vi "Pump_API_ForceMonitoring_Test.vi"() -> ()   [LabVIEW 2010]
uses:
  labbCAN_Bus_API/labbCAN_Bus_API.lvlib
  labbCAN_Pump_API/labbCAN_Pump_API.lvlib
panel:
  out "Force Plot":dbl(graph)
  out "Safety Stop Active":bool
  out "Force":dbl
  out "Flow":dbl
  out "Force Monitoring Enabled":bool
  out "Position Sensing Initialized":bool
  out "Status":string="Test 5: Continuous flow dosage"
  out "Test Step:":string
  out "error out":errorcluster
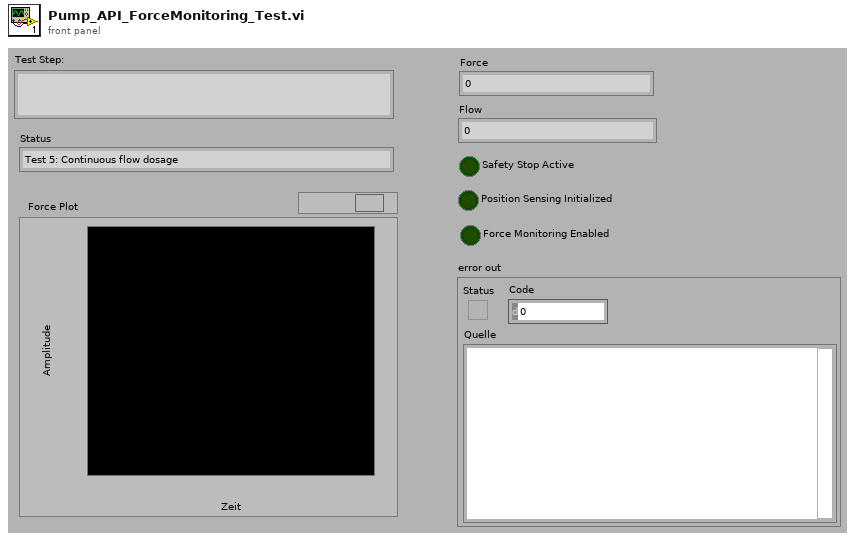
[diagram p1: front panel]
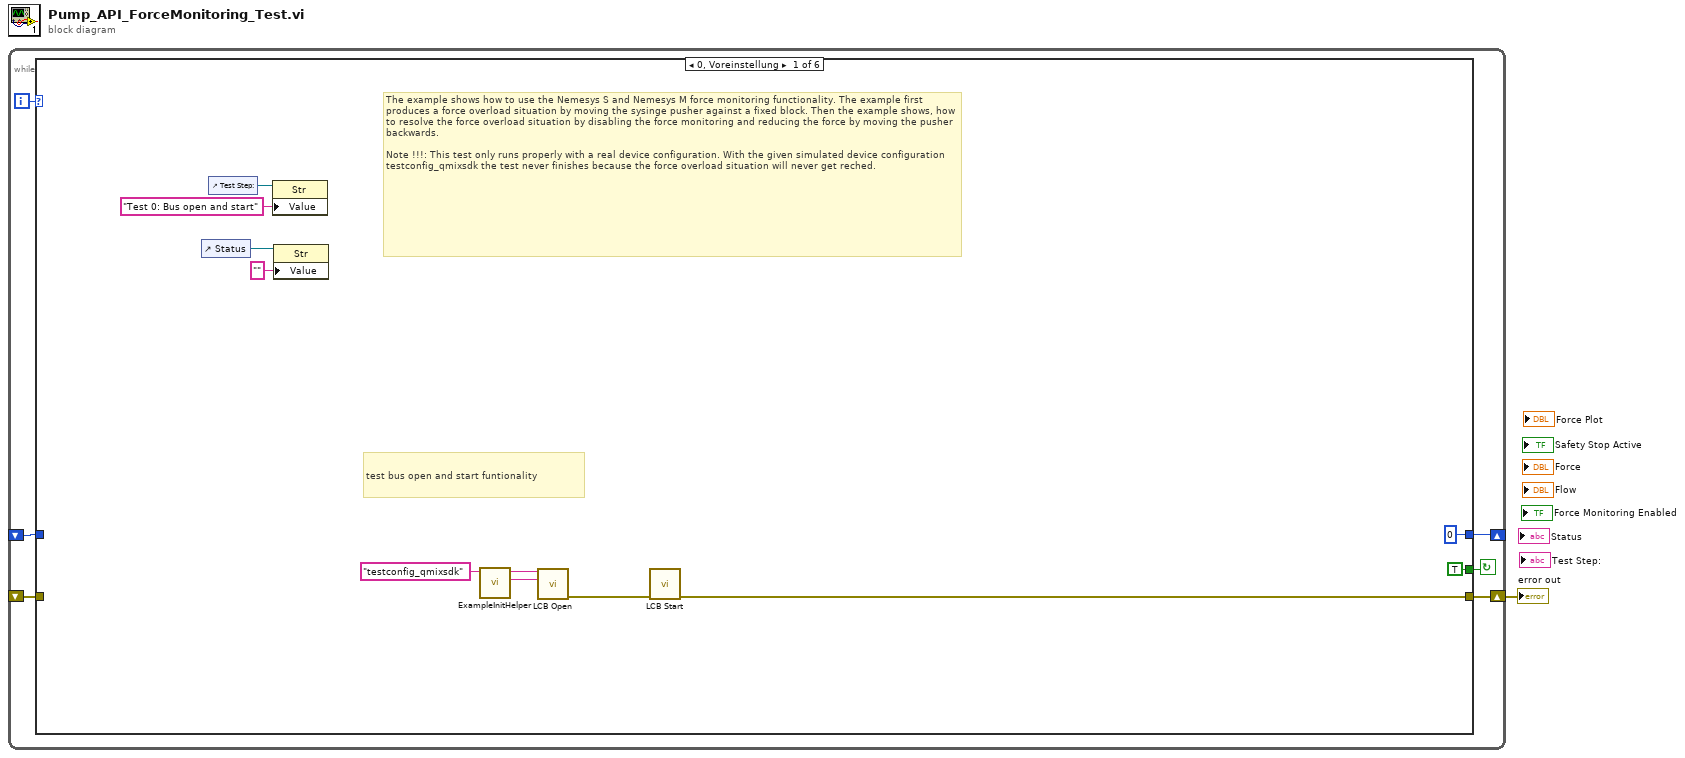
[diagram p0: block diagram]
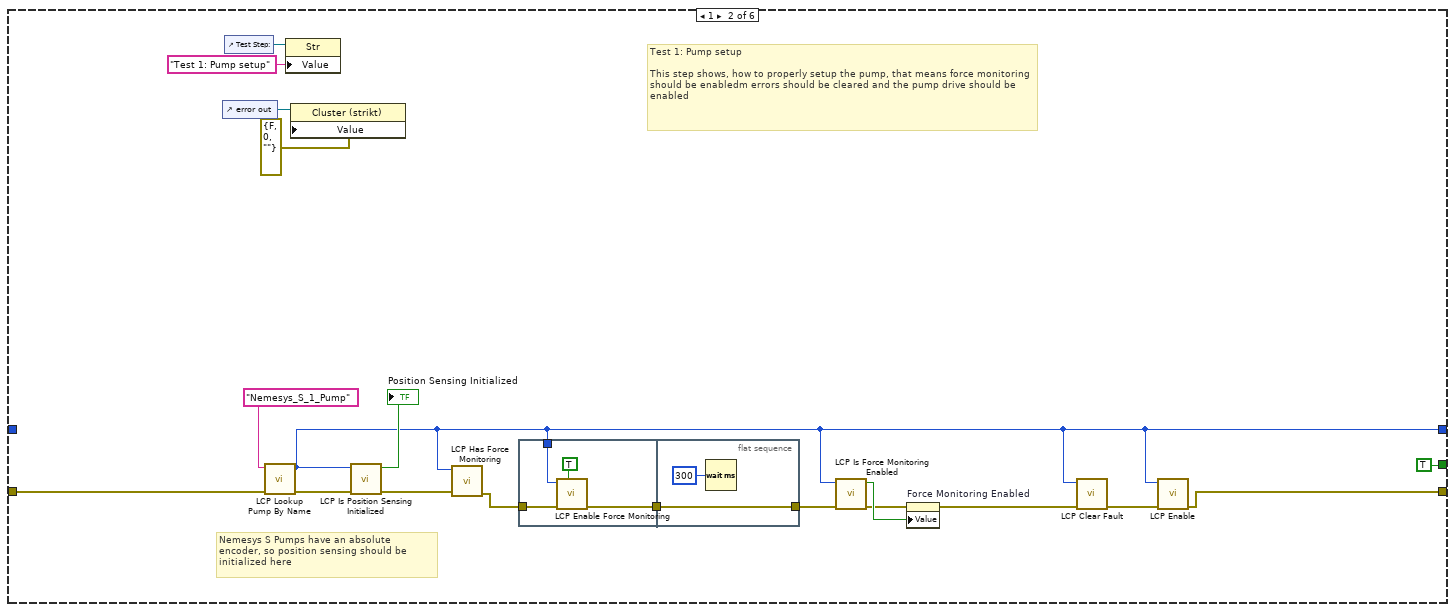
[diagram p2: hidden frame]
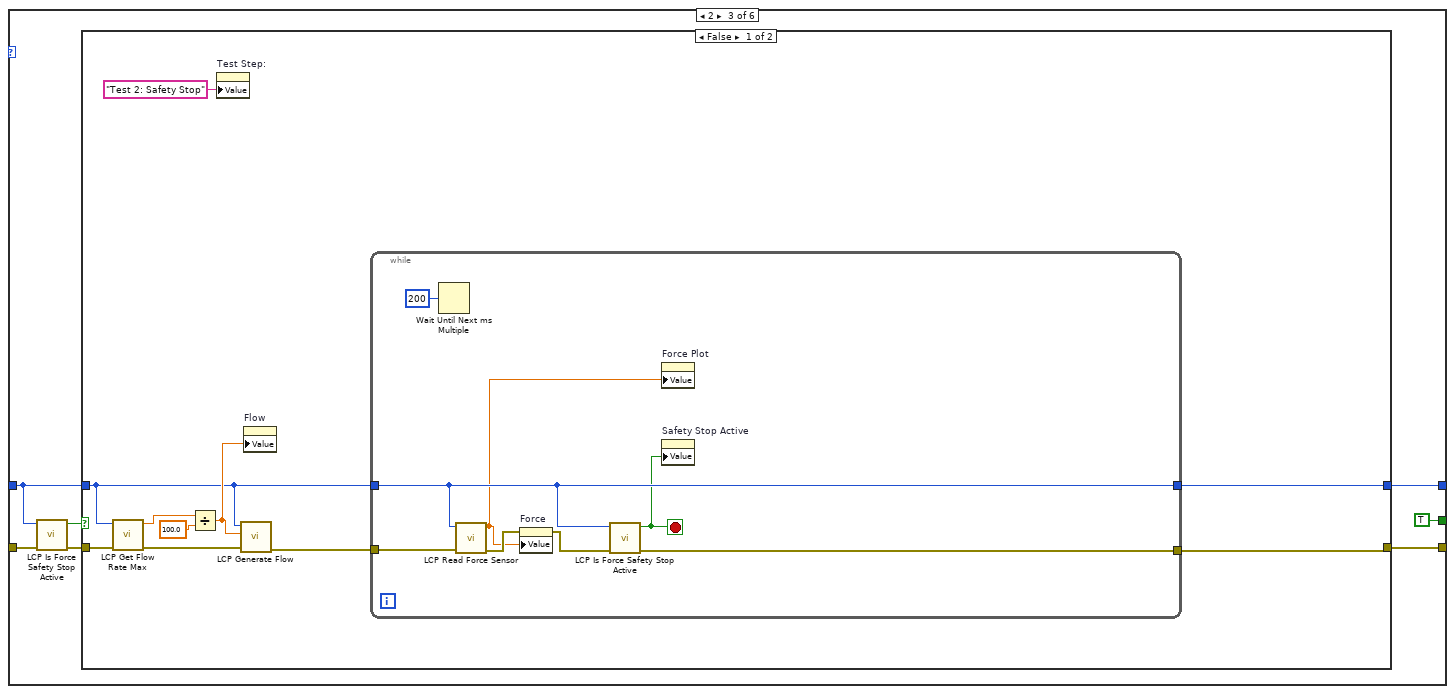
[diagram p3: hidden frame]
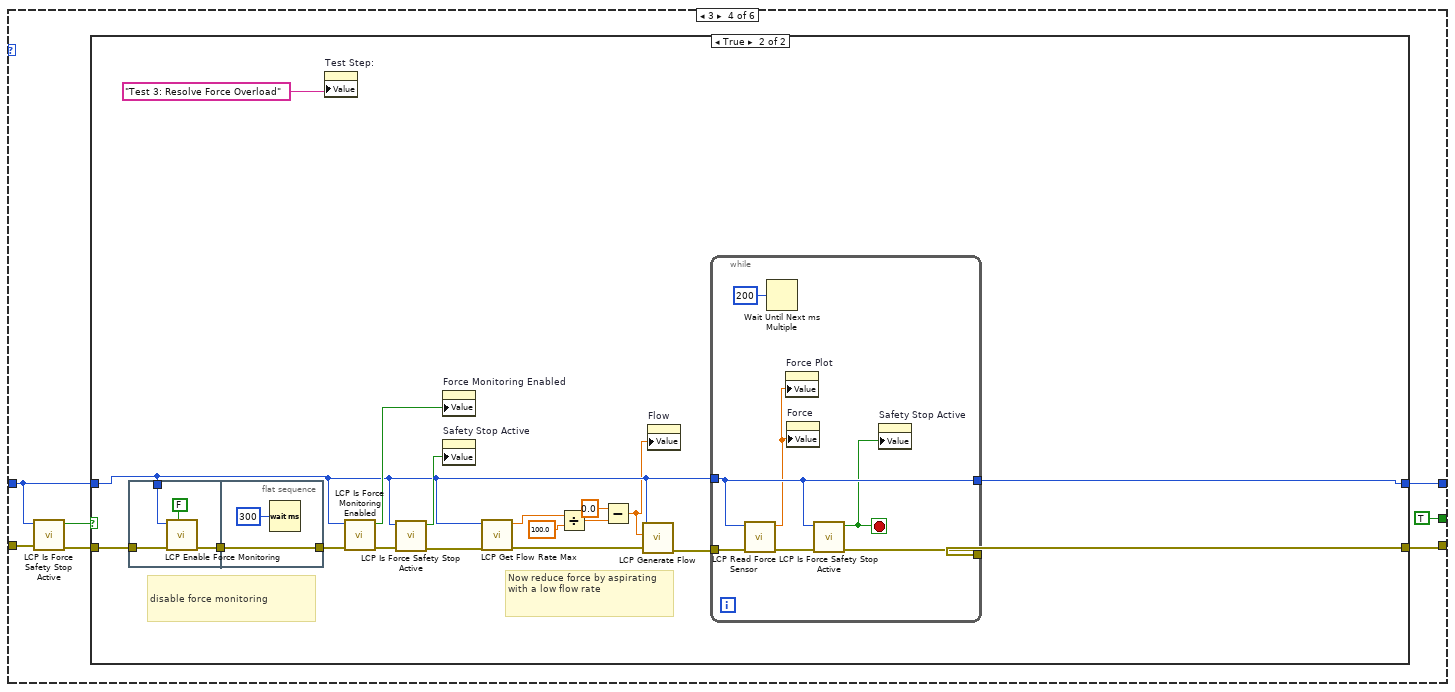
[diagram p5: hidden frame]
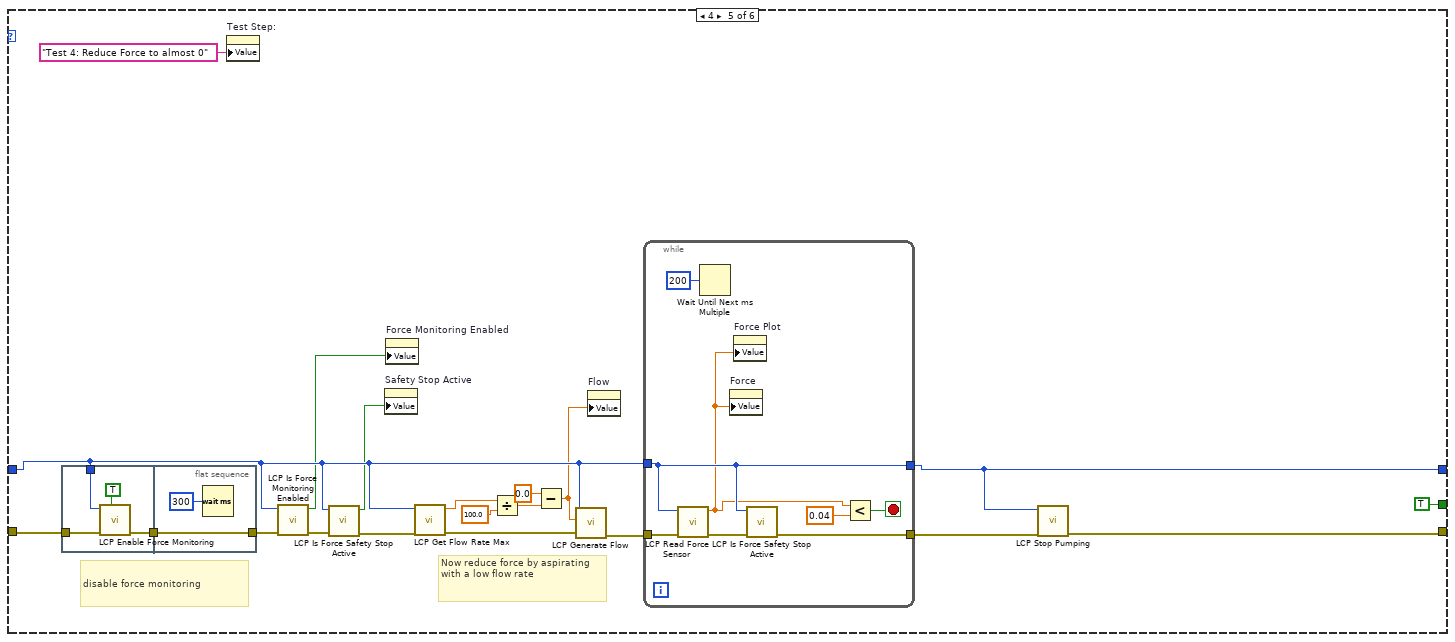
[diagram p7: hidden frame]
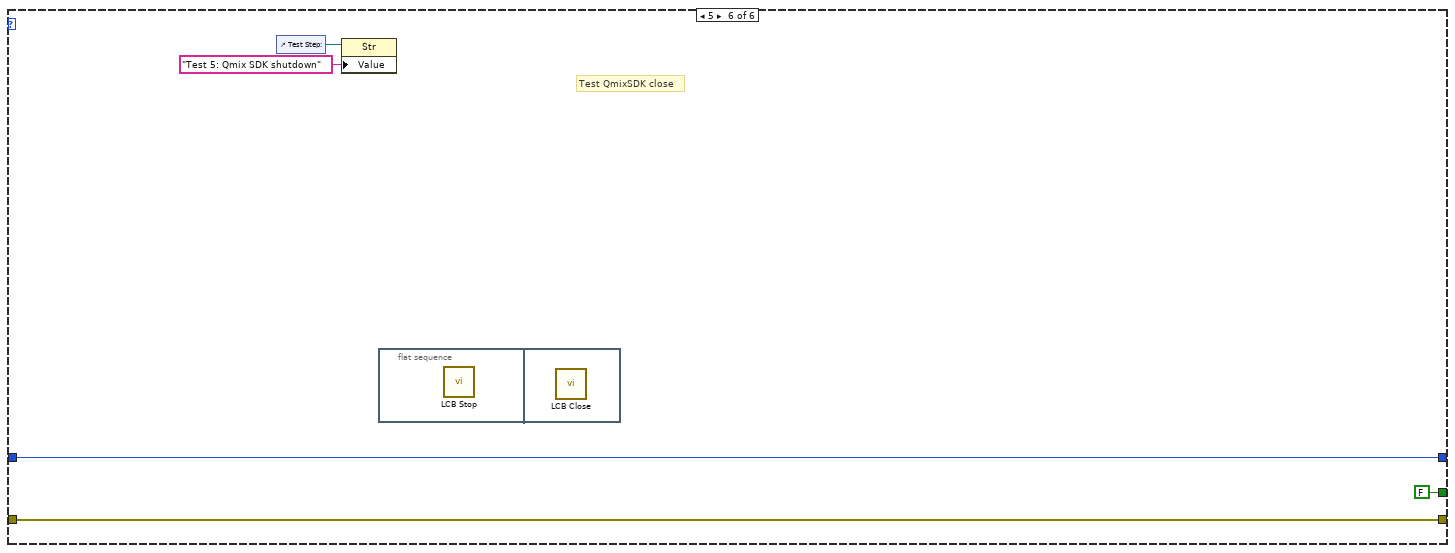
[diagram p8: hidden frame]
diagram:
  n1 = while {
    shift-right: [w2] -> w1
    shift-left: _ -> [w5]
    shift-right: [w4] -> _
    shift-left: _ -> [w3]
    i -> [w7]
    stop <- w6 continue-if-true
    n2 = case shown="0, Voreinstellung" w7 {
      tunnel: [TRUE TRUE TRUE TRUE TRUE FALSE] -> w6
      tunnel: w5 -> [_ w35 w49 w77 w119 w145]
      tunnel: [w16 w19 w46 w75 w112 w145] -> w2
      tunnel: [i64 0 ("ContiFlowPumpHandle") w20 w44 w71 w111 w148] -> w4
      tunnel: w3 -> [_ _ w45 w72 w118 w148]
      frame 0, Default {
        # "The example shows how to use the Nemesys S and Nemesys M force monitoring functionality. The example first produces a force overload situation by moving the sysinge pusher against a fixed block. Then the example shows, how to resolve the force overload situation by disabling the force monitoring and reducing the force by moving the pusher backwards.\n\nNote !!!: This test only runs properly with a real device configuration. With the given simulated device configuration testconfig_qmixsdk the test never finishes because the force overload situation will never get reched."
        # "test bus open and start funtionality"
        n3 = control-ref of="Status"() -> (w12:refnum<vi>)
        n4 = control-ref of="Test Step:"() -> (w14:refnum<vi>)
        n5 = property class="Str"(reference=w14, "Value"="Test 0: Bus open and start" ("Wert")) -> ()  [unwired: 1 in, 2 out]
        n6 = property class="Str"(reference=w12, "Value"="" ("Wert")) -> ()  [unwired: 1 in, 2 out]
        n7 = call "ExampleInitHelper.vi"("Device Config Name"="testconfig_qmixsdk") -> ("Plugin Search Path"=w9:string, "Device Configuration Path"=w10:string)  [unwired: 5 in]
        n8 = call "LCB Open.vi"("PluginSearchPath"=w9, "Device Configuration Path"=w10) -> ("error out"=w17:errorcluster)  [unwired: 9 in]
        n9 = call "LCB Start.vi"("error in (no error)"=w17) -> ("error out"=w16:errorcluster)  [unwired: 10 in]
      }
      frame 1 {
        # "Nemesys S Pumps have an absolute encoder, so position sensing should be initialized here"
        # "Test 1: Pump setup\n\nThis step shows, how to properly setup the pump, that means force monitoring should be enabledm errors should be cleared and the pump drive should be enabled"
        n10 = control-ref of="error out"() -> (w32:refnum<vi>)
        n11 = control-ref of="Test Step:"() -> (w34:refnum<vi>)
        n12 = call "LCP Lookup Pump By Name.vi"("error in (no error)"=w35, "Pump Name"="Nemesys_S_1_Pump" ("pAxisName")) -> ("error out"=w30:errorcluster, "Pump handle"=w20:i64)  [unwired: 8 in]
        n13 = property class="Str"(reference=w34, "Value"="Test 1: Pump setup" ("Wert")) -> ()  [unwired: 1 in, 2 out]
        n14 = property class="Cluster (strikt)"(reference=w32, "Value"=errorcluster {"status"=FALSE, "code"=0, "source"=""} ("Wert")) -> ()  [unwired: 1 in, 2 out]
        n15 = call "LCP Is Position Sensing Initialized.vi"("error in (no error)"=w30, "Pump Handle"=w20) -> ("error out"=w28:errorcluster, "Initialized"=→"Position Sensing Initialized":bool)  [unwired: 8 in]
        n16 = call "LCP Has Force Monitoring.vi"("error in (no error)"=w28, "Pump Handle"=w20) -> ("error out"=w27:errorcluster)  [unwired: 8 in, 1 out]
        n17 = flat-sequence {
          tunnel: w27 -> [w40]
          tunnel: w20 -> [w39]
          tunnel: [w38] -> w26
          tunnel: [w42] -> w25
          tunnel: w26 -> [w42]
          frame #0 {
            n18 = call "LCP Enable Force Monitoring.vi"("Enable"=TRUE, "error in (no error)"=w40, "Pump Handle"=w39) -> ("error out"=w38:errorcluster)  [unwired: 8 in]
          }
          frame #1 {
            n19 = Wait (ms)(milliseconds to wait=u32 300 ("Zu wartende ms")) -> ()  [unwired: 1 out]
          }
        }
        n20 = call "LCP Is Force Monitoring Enabled.vi"("error in (no error)"=w25, "Pump Handle"=w20) -> ("error out"=w23:errorcluster, "Force Monitoring Enabled"=w24:bool)  [unwired: 8 in]
        n21 = property on="Force Monitoring Enabled" class="Bool. (strikt)"(error in=w23, "Value"=w24) -> (error out=w22:errorcluster)  [unwired: 1 in, 1 out]
        n22 = call "LCP Clear Fault.vi"("error in (no error)"=w22, "Pump Handle"=w20) -> ("error out"=w21:errorcluster)  [unwired: 9 in]
        n23 = call "LCP Enable.vi"("error in (no error)"=w21, "Pump Handle"=w20) -> ("error out"=w19:errorcluster)  [unwired: 9 in]
      }
      frame 2 {
        n24 = call "LCP Is Force Safety Stop Active.vi"("error in (no error)"=w49, "Pump Handle"=w45) -> ("error out"=w47:errorcluster, "Safety Stop Active"=w48:bool)  [unwired: 8 in]
        n25 = case shown="False" w48 {
          tunnel: w47 -> [w59 w70]
          tunnel: [w52 w70] -> w46
          tunnel: w45 -> [w53 w69]
          tunnel: [w51 w69] -> w44
          frame False {
            n26 = call "LCP Get Flow Rate Max.vi"("error in (no error)"=w59, "Pump Handle"=w53) -> ("error out"=w56:errorcluster, "Maximum Flow Rate"=w58:dbl)  [unwired: 8 in]
            n27 = Divide(x=w58, y=100.0) -> (x/y=w55:dbl)
            n28 = property on="Test Step:" class="Str"("Value"="Test 2: Safety Stop" ("Test Step:")) -> ()  [unwired: 2 in, 2 out]
            n29 = call "LCP Generate Flow.vi"("error in (no error)"=w56, "Flow Rate"=w55, "Pump Handle"=w53) -> ("error out"=w54:errorcluster)  [unwired: 8 in]
            n30 = property on="Flow" class="DigWert (strikt)"("Value"=w55) -> ()  [unwired: 2 in, 2 out]
            n31 = while {
              tunnel: w54 -> [w67]
              tunnel: w53 -> [w63]
              tunnel: [w64] -> w52
              tunnel: [w63] -> w51
              stop <- w62 stop-if-true
              n32 = Wait Until Next ms Multiple(millisecond multiple=u32 200 ("Vielfache von ms")) -> ()  [unwired: 1 out]
              n33 = call "LCP Read Force Sensor.vi"("error in (no error)"=w67, "Pump Handle"=w63) -> ("error out"=w66:errorcluster, "Force"=w61:dbl)  [unwired: 8 in]
              n34 = property on="Force" class="DigWert (strikt)"(error in=w66, "Value"=w61) -> (error out=w65:errorcluster)  [unwired: 1 in, 1 out]
              n35 = call "LCP Is Force Safety Stop Active.vi"("error in (no error)"=w65, "Pump Handle"=w63) -> ("error out"=w64:errorcluster, "Safety Stop Active"=w62:bool)  [unwired: 8 in]
              n36 = property on="Force Plot" class="SVDiagr (strikt)"("Value"=w61) -> ()  [unwired: 2 in, 2 out]
              n37 = property on="Safety Stop Active" class="Bool. (strikt)"("Value"=w62) -> ()  [unwired: 2 in, 2 out]
            }
          }
          frame True {
          }
        }
      }
      frame 3 {
        n38 = call "LCP Is Force Safety Stop Active.vi"("error in (no error)"=w77, "Pump Handle"=w72) -> ("error out"=w76:errorcluster, "Safety Stop Active"=w73:bool)  [unwired: 8 in]
        n39 = case shown="True" w73 {
          tunnel: [w79 w83] -> w75
          tunnel: w76 -> [w79 w93]
          tunnel: w72 -> [w78 w84]
          tunnel: [w78 w82] -> w71
          frame False {
          }
          frame True {
            # "disable force monitoring"
            # "Now reduce force by aspirating with a low flow rate"
            n40 = flat-sequence {
              tunnel: w84 -> [w100]
              tunnel: w93 -> [w99]
              tunnel: [w98] -> w92
              tunnel: [w102] -> w91
              tunnel: w92 -> [w102]
              frame #0 {
                n41 = call "LCP Enable Force Monitoring.vi"("Enable"=FALSE, "error in (no error)"=w99, "Pump Handle"=w100) -> ("error out"=w98:errorcluster)  [unwired: 8 in]
              }
              frame #1 {
                n42 = Wait (ms)(milliseconds to wait=u32 300 ("Zu wartende ms")) -> ()  [unwired: 1 out]
              }
            }
            n43 = property on="Test Step:" class="Str"("Value"="Test 3: Resolve Force Overload" ("Test Step:")) -> ()  [unwired: 2 in, 2 out]
            n44 = call "LCP Is Force Monitoring Enabled.vi"("error in (no error)"=w91, "Pump Handle"=w84) -> ("error out"=w90:errorcluster, "Force Monitoring Enabled"=w89:bool)  [unwired: 8 in]
            n45 = call "LCP Is Force Safety Stop Active.vi"("error in (no error)"=w90, "Pump Handle"=w84) -> ("error out"=w87:errorcluster, "Safety Stop Active"=w88:bool)  [unwired: 8 in]
            n46 = property on="Force Monitoring Enabled" class="Bool. (strikt)"("Value"=w89) -> ()  [unwired: 2 in, 2 out]
            n47 = property on="Safety Stop Active" class="Bool. (strikt)"("Value"=w88) -> ()  [unwired: 2 in, 2 out]
            n48 = call "LCP Get Flow Rate Max.vi"("error in (no error)"=w87, "Pump Handle"=w84) -> ("error out"=w95:errorcluster, "Maximum Flow Rate"=w97:dbl)  [unwired: 8 in]
            n49 = Divide(x=w97, y=100.0) -> (x/y=w86:dbl)
            n50 = Subtract(x=0.0, y=w86) -> (x-y=w80:dbl)
            n51 = call "LCP Generate Flow.vi"("error in (no error)"=w95, "Flow Rate"=w80, "Pump Handle"=w84) -> ("error out"=w94:errorcluster)  [unwired: 8 in]
            n52 = property on="Flow" class="DigWert (strikt)"("Value"=w80) -> ()  [unwired: 2 in, 2 out]
            n53 = while {
              tunnel: w94 -> [w109]
              tunnel: [w108] -> w83
              tunnel: w84 -> [w106]
              tunnel: [w106] -> w82
              stop <- w105 stop-if-true
              n54 = call "LCP Read Force Sensor.vi"("error in (no error)"=w109, "Pump Handle"=w106) -> ("error out"=w107:errorcluster, "Force"=w104:dbl)  [unwired: 8 in]
              n55 = Wait Until Next ms Multiple(millisecond multiple=u32 200 ("Vielfache von ms")) -> ()  [unwired: 1 out]
              n56 = property on="Force Plot" class="SVDiagr (strikt)"("Value"=w104) -> ()  [unwired: 2 in, 2 out]
              n57 = property on="Force" class="DigWert (strikt)"("Value"=w104) -> ()  [unwired: 2 in, 2 out]
              n58 = call "LCP Is Force Safety Stop Active.vi"("error in (no error)"=w107, "Pump Handle"=w106) -> ("error out"=w108:errorcluster, "Safety Stop Active"=w105:bool)  [unwired: 8 in]
              n59 = property on="Safety Stop Active" class="Bool. (strikt)"("Value"=w105) -> ()  [unwired: 2 in, 2 out]
            }
          }
        }
      }
      frame 4 {
        # "disable force monitoring"
        # "Now reduce force by aspirating with a low flow rate"
        n60 = flat-sequence {
          tunnel: w118 -> [w133]
          tunnel: w119 -> [w132]
          tunnel: [w131] -> w129
          tunnel: [w135] -> w124
          tunnel: w129 -> [w135]
          frame #0 {
            n61 = call "LCP Enable Force Monitoring.vi"("Enable"=TRUE, "error in (no error)"=w132, "Pump Handle"=w133) -> ("error out"=w131:errorcluster)  [unwired: 8 in]
          }
          frame #1 {
            n62 = Wait (ms)(milliseconds to wait=u32 300 ("Zu wartende ms")) -> ()  [unwired: 1 out]
          }
        }
        n63 = property on="Test Step:" class="Str"("Value"="Test 4: Reduce Force to almost 0" ("Test Step:")) -> ()  [unwired: 2 in, 2 out]
        n64 = call "LCP Is Force Monitoring Enabled.vi"("error in (no error)"=w124, "Pump Handle"=w118) -> ("error out"=w123:errorcluster, "Force Monitoring Enabled"=w117:bool)  [unwired: 8 in]
        n65 = call "LCP Is Force Safety Stop Active.vi"("error in (no error)"=w123, "Pump Handle"=w118) -> ("error out"=w122:errorcluster, "Safety Stop Active"=w116:bool)  [unwired: 8 in]
        n66 = property on="Safety Stop Active" class="Bool. (strikt)"("Value"=w116) -> ()  [unwired: 2 in, 2 out]
        n67 = property on="Force Monitoring Enabled" class="Bool. (strikt)"("Value"=w117) -> ()  [unwired: 2 in, 2 out]
        n68 = call "LCP Get Flow Rate Max.vi"("error in (no error)"=w122, "Pump Handle"=w118) -> ("error out"=w126:errorcluster, "Maximum Flow Rate"=w128:dbl)  [unwired: 8 in]
        n69 = Divide(x=w128, y=100.0) -> (x/y=w121:dbl)
        n70 = Subtract(x=0.0, y=w121) -> (x-y=w115:dbl)
        n71 = call "LCP Generate Flow.vi"("error in (no error)"=w126, "Flow Rate"=w115, "Pump Handle"=w118) -> ("error out"=w125:errorcluster)  [unwired: 8 in]
        n72 = property on="Flow" class="DigWert (strikt)"("Value"=w115) -> ()  [unwired: 2 in, 2 out]
        n73 = while {
          tunnel: w125 -> [w143]
          tunnel: [w142] -> w113
          tunnel: w118 -> [w140]
          tunnel: [w140] -> w111
          stop <- w139 stop-if-true
          n74 = call "LCP Read Force Sensor.vi"("error in (no error)"=w143, "Pump Handle"=w140) -> ("error out"=w141:errorcluster, "Force"=w137:dbl)  [unwired: 8 in]
          n75 = Wait Until Next ms Multiple(millisecond multiple=u32 200 ("Vielfache von ms")) -> ()  [unwired: 1 out]
          n76 = property on="Force" class="DigWert (strikt)"("Value"=w137) -> ()  [unwired: 2 in, 2 out]
          n77 = property on="Force Plot" class="SVDiagr (strikt)"("Value"=w137) -> ()  [unwired: 2 in, 2 out]
          n78 = call "LCP Is Force Safety Stop Active.vi"("error in (no error)"=w141, "Pump Handle"=w140) -> ("error out"=w142:errorcluster)  [unwired: 8 in, 1 out]
          n79 = Less?(x=w137, y=0.04) -> (x < y?=w139:bool)
        }
        n80 = call "LCP Stop Pumping.vi"("error in (no error)"=w113, "Pump Handle"=w111) -> ("error out"=w112:errorcluster)  [unwired: 9 in]
      }
      frame 5 {
        # "Test QmixSDK close"
        n81 = control-ref of="Test Step:"() -> (w147:refnum<vi>)
        n82 = property class="Str"(reference=w147, "Value"="Test 5: Qmix SDK shutdown" ("Wert")) -> ()  [unwired: 1 in, 2 out]
        n83 = flat-sequence {
          frame #0 {
            n84 = call "LCB Stop.vi"() -> ()  [unwired: 11 in, 1 out]
          }
          frame #1 {
            n85 = call "LCB Close.vi"() -> ()  [unwired: 11 in, 1 out]
          }
        }
      }
    }
  }
  "error out" <- w1
